vi "Cluster-Find.vi"() -> ()   [LabVIEW 2018]
uses:
  <vilib>/Platform/TimedLoop/XDataNode/timing_clust.ctl
  <vilib>/Platform/TimedLoop/XDataNode/nitl_modes.ctl
  <vilib>/Platform/TimedLoop/XDataNode/wakeup.ctl
  <vilib>/rvi/Emulation/niFpgaSctlEmulationGetInTimedLoop.vi
  <vilib>/rvi/Emulation/niFpgaEmulationReportErrorSimple.vi
  <vilib>/rvi/Emulation/niFpgaGetClockAttributes.vi
  <vilib>/rvi/Emulation/niFpgaCriticalErrorInLSC.vi
  <vilib>/rvi/eio/common/nirviEmuTemplateMethod_errors.vi
  <vilib>/Platform/TimedLoop/XDataNode/XDataNode.xnode
  <vilib>/eio/EIONode/EIONode.xnode
  <vilib>/Platform/TimedLoop/XDataNode/XDNodeRunTimeDep.lvlib
panel:
  out "1":bool[](array[boolean])
  out "2":bool[](array[boolean])
  out "3":bool[](array[boolean])
  out "Nontrivial":i16
  out "4":bool[](array[boolean])
  out "04":i16
  out "03":i16
  out "02":i16
  out "01":i16
  out "clock2":i16
  out "4":i16
  out "3":i16
  out "2":i16
  out "1":i16
  out "Final":bool
  out "2V-ad":bool
  out "2H-ad":bool
  out "1V-ad":bool
  out "1H-ad":bool
  out "SE_Ch4_Rd":bool
  out "SE_Ch3_Rd":bool
  out "SE_Ch2_Rd":bool
  out "SE_Ch1_Rd":bool
  out "clock1":i16
  out "Test":bool
  in  "Probing-Depth":i16
  in  "Stop Button":bool
  in  "2V":i16
  in  "1V":i16
  in  "2H":i16
  in  "1H":i16
  out "Round":u32 format="%^.0e"
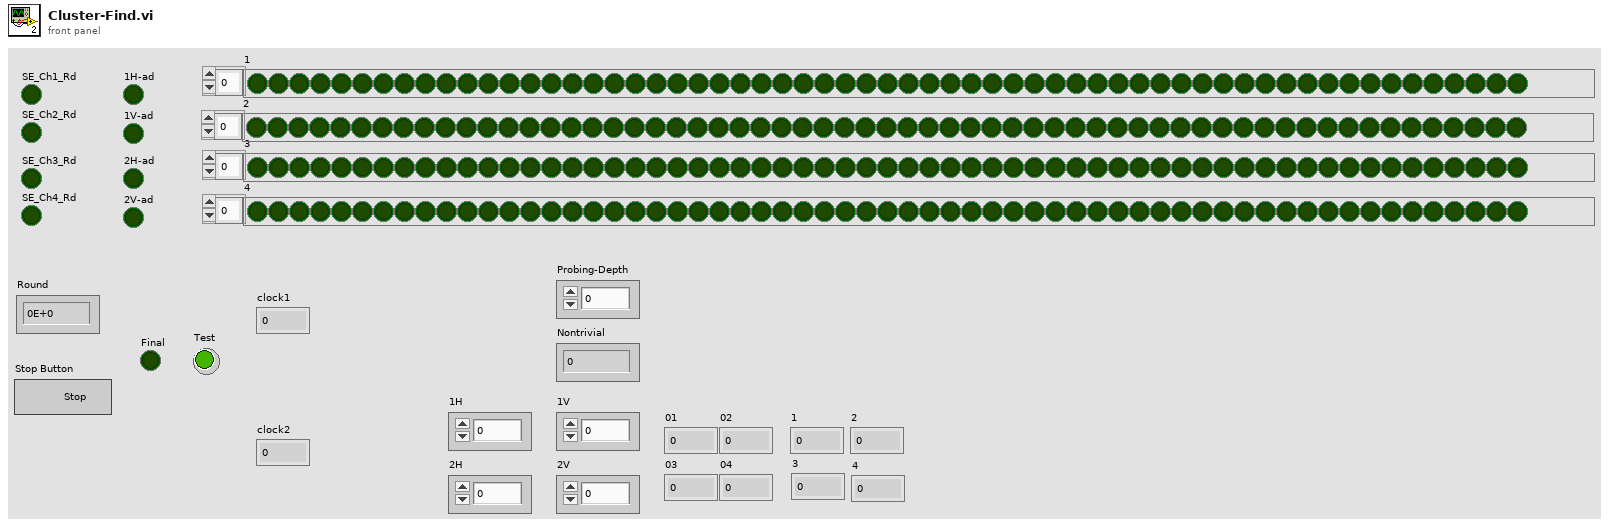
[diagram p1: front panel]
types:
  T1 = typedef "XDNodeRunTimeDep.lvlib/timing_clust.ctl" = cluster{"Expected End [f-1]":u64, "Actual End [f-1]":u64, "Finished Late? [f-1]":bool, "Expected End [i-1]":u64, "Actual End [i-1]":u64, "Finished Late? [i-1]":bool, "Expected Start [i]":u64, "Actual Start [i]":u64, "Expected Start [f]":u64, "Actual Start [f]":u64, "Source Name":string, "Structure Name":string, "Period":i64, "Deadline":i64, "Offset":i64, "Start":i64, "Priority":i32, "Timeout":i32, "Mode":T2, "Wakeup Reason":T3, "Error":errorcluster, "Source Type":string, "Secondary Source Type":string, "Global End Time":u64, "Global Start Time":u64, "Frame Duration":u64, "Iteration Duration":u64, "Assigned CPU":i32, "I/O Scan Engine Mode":u32}
  T2 = typedef "XDNodeRunTimeDep.lvlib/nitl_modes.ctl" = enum32{"No Change", "Process missed periods, maintain original phase", "Discard missed periods, maintain original phase", "Process missed periods, ignore original phase", "Discard missed periods, ignore original phase"}
  T3 = typedef "XDNodeRunTimeDep.lvlib/wakeup.ctl" = enum32{"Normal", "Aborted", "Asynchronous wakeup", "Timing source error", "Timed loop error", "Timeout"}
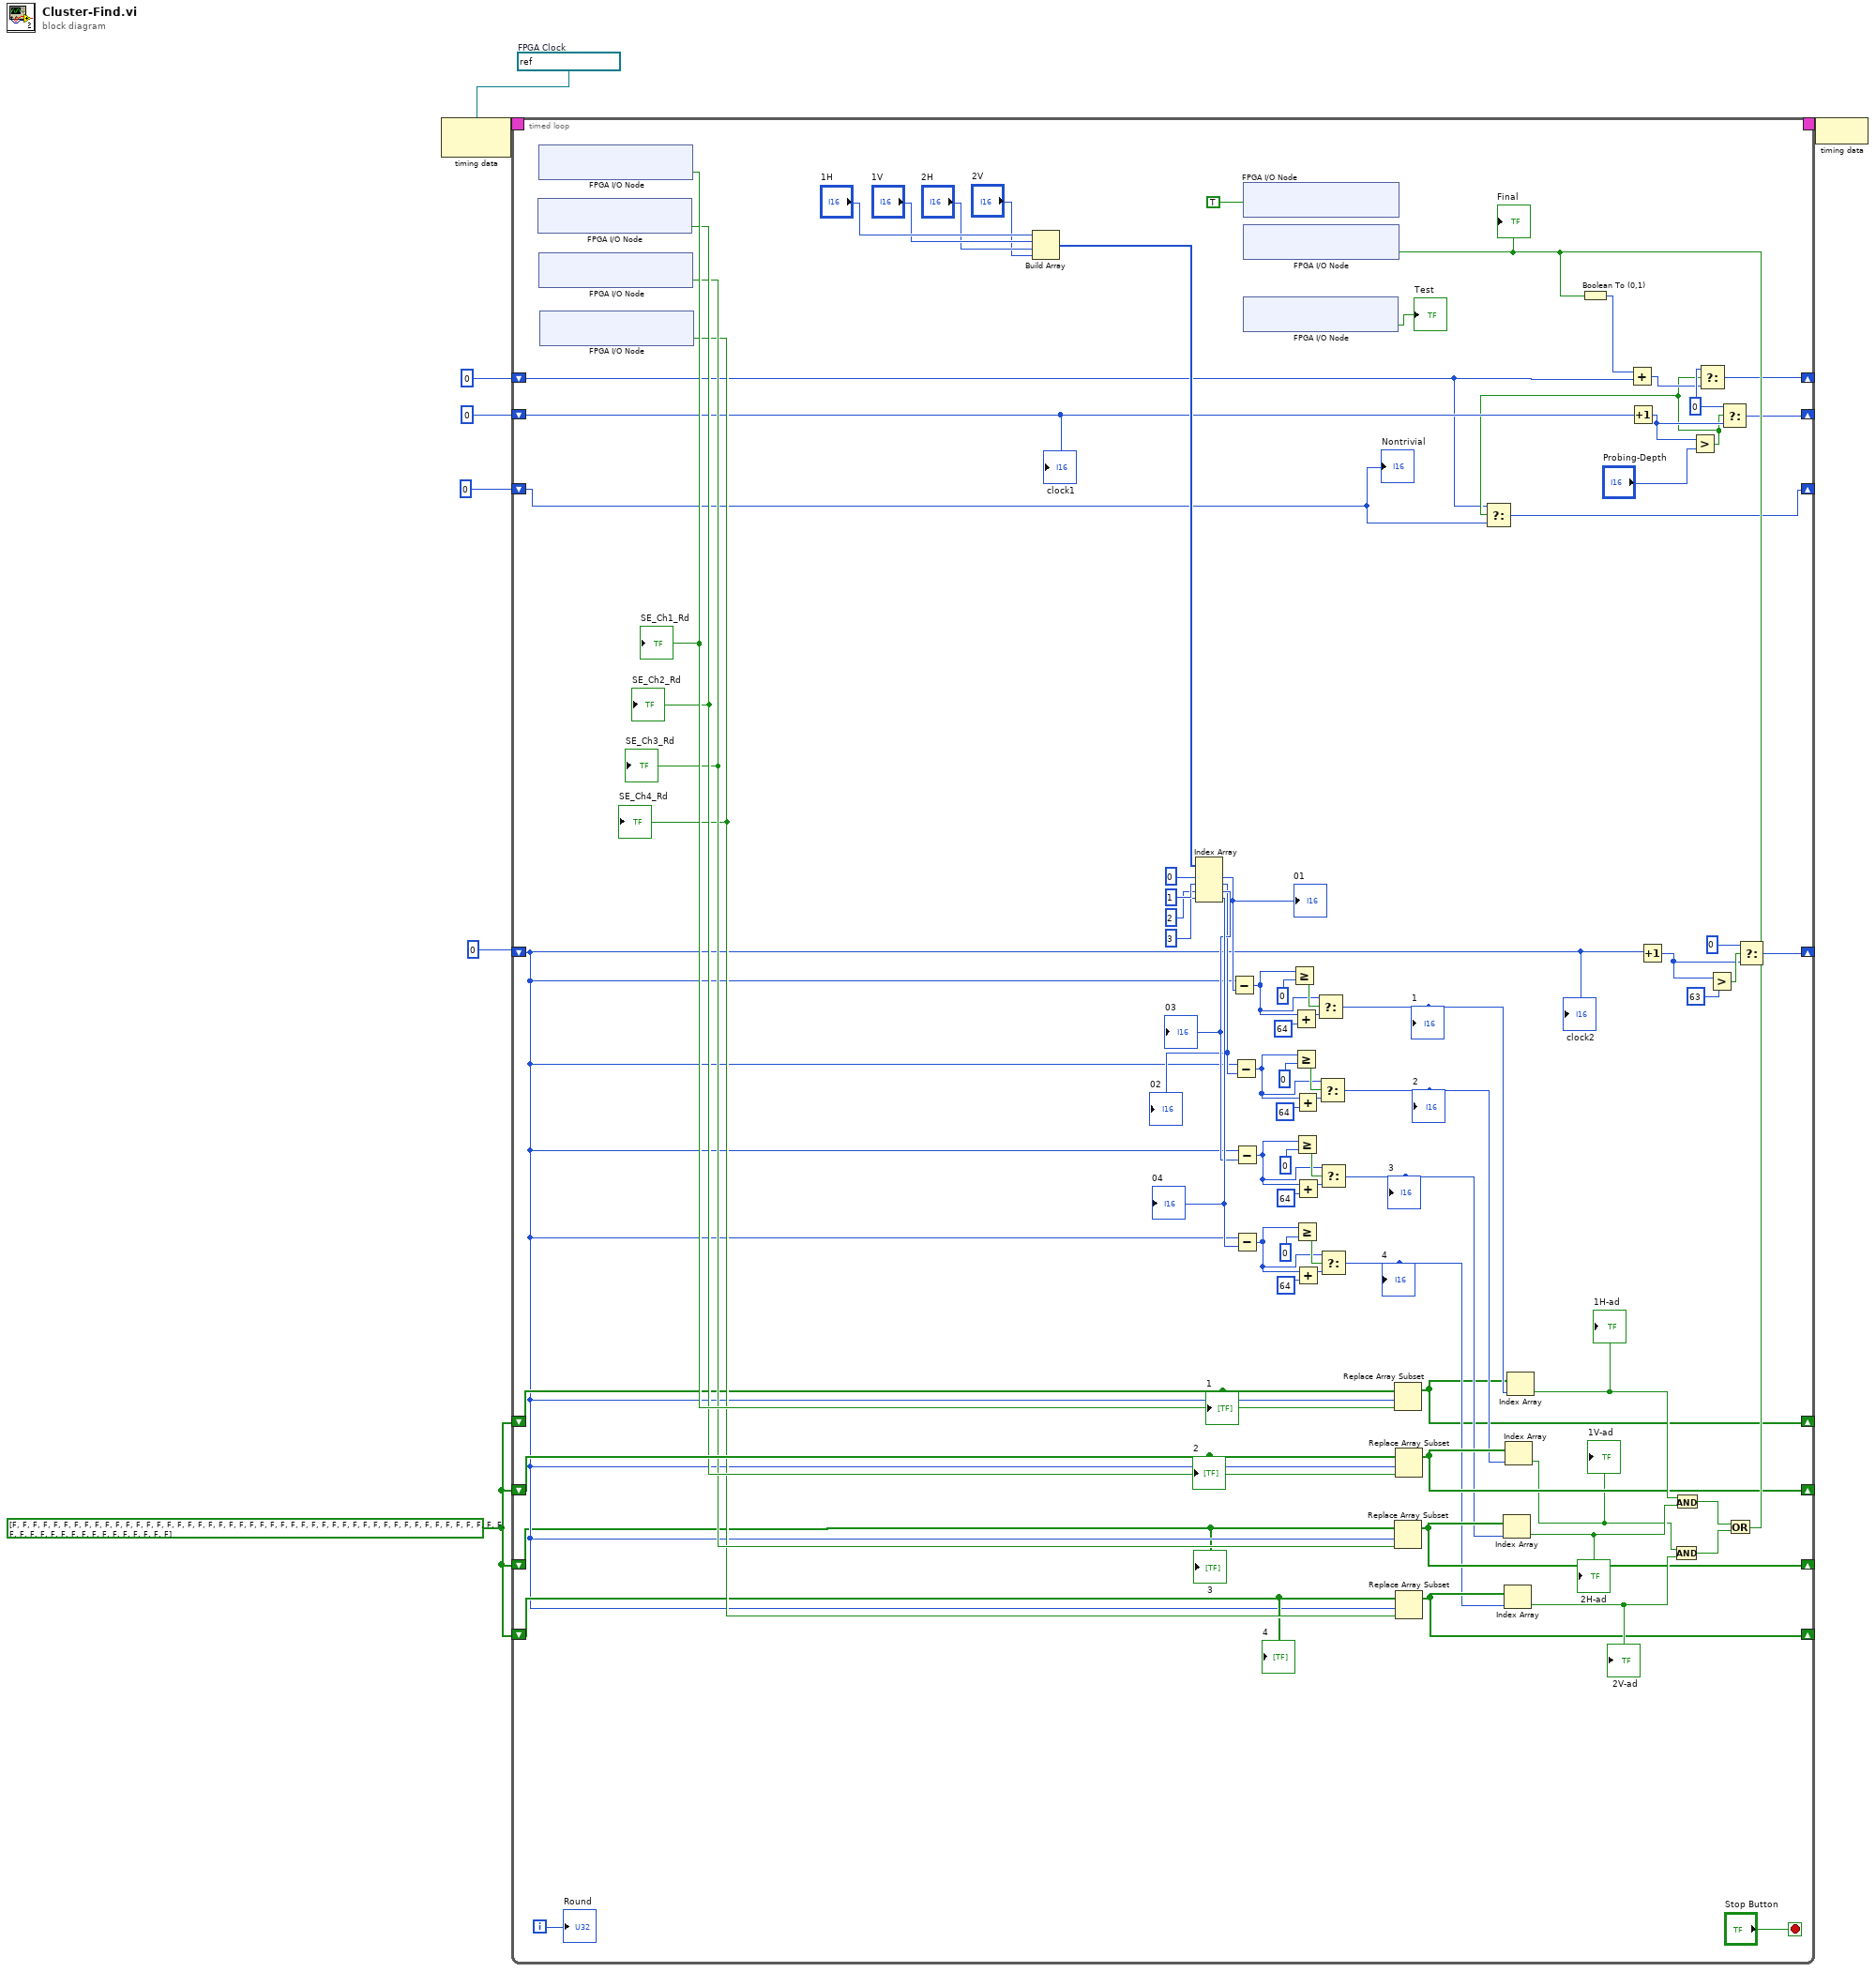
[diagram p0: block diagram]
diagram:
  w5 = bool[] [FALSE, FALSE, FALSE, FALSE, FALSE, FALSE, FALSE, FALSE, FALSE, FALSE, FALSE, FALSE, FALSE, FALSE, FALSE, FALSE, FALSE, FALSE, FALSE, FALSE, FALSE, FALSE, FALSE, FALSE, FALSE, FALSE, FALSE, FALSE, FALSE, FALSE, FALSE, FALSE, FALSE, FALSE, FALSE, FALSE, FALSE, FALSE, FALSE, FALSE, FALSE, FALSE, FALSE, FALSE, FALSE, FALSE, FALSE, FALSE, FALSE, FALSE, FALSE, FALSE, FALSE, FALSE, FALSE, FALSE, FALSE, FALSE, FALSE, FALSE, FALSE, FALSE, FALSE, FALSE]
  w6 = refnum<k21> "200 MHz Clock"  # FPGA Clock
  n1 = node-c288(w6) -> (w8:T1)
  n2 = timed-loop {
    timing: w8 -> [_]
    timing-out: [_] -> w7
    shift-right: [w19] -> _
    shift-left: w5 -> [w15]
    shift-right: [w72] -> _
    shift-left: w5 -> [w73]
    shift-right: [w70] -> _
    shift-left: w5 -> [w13]
    shift-right: [w68] -> _
    shift-left: w5 -> [w16]
    shift-right: [w74] -> _
    shift-left: i16 0 -> [w14]
    shift-right: [w32] -> _
    shift-left: i16 0 -> [w26]
    shift-right: [w27] -> _
    shift-left: i16 0 -> [w10]
    shift-right: [w11] -> _
    shift-left: i16 0 -> [w9]
    i -> [w83]
    stop <- "Stop Button" stop-if-true
    w29 = i16 0
    n3 = xnode "FPGA I/O Node"() -> ("IO Module\\SE_Ch2_Rd"=w71:bool)  [unwired: 1 in, 1 out]
    "SE_Ch2_Rd" <- w71
    n4 = xnode "FPGA I/O Node"() -> ("IO Module\\SE_Ch1_Rd"=w78:bool)  [unwired: 1 in, 1 out]
    "SE_Ch1_Rd" <- w78
    n5 = xnode "FPGA I/O Node"() -> ("IO Module\\SE_Ch3_Rd"=w69:bool)  [unwired: 1 in, 1 out]
    "SE_Ch3_Rd" <- w69
    n6 = xnode "FPGA I/O Node"() -> ("IO Module\\SE_Ch4_Rd"=w67:bool)  [unwired: 1 in, 1 out]
    "SE_Ch4_Rd" <- w67
    n7 = Build Array("1H", "1V", "2H", "2V") -> (w61:i16[])
    n8 = Index Array(array=w61, index #1=i16 0, index #2=i16 1, index #3=i16 2, index #4=i16 3) -> (element #1=w59:i16, element #2=w17:i16, element #3=w18:i16, element #4=w38:i16)
    "01" <- w59
    "02" <- w17
    "03" <- w18
    "04" <- w38
    n9 = Subtract(x=w14, y=w59) -> (x-y=w23:i16)
    n10 = Subtract(x=w14, y=w17) -> (x-y=w22:i16)
    n11 = Subtract(x=w14, y=w18) -> (x-y=w21:i16)
    n12 = Subtract(x=w14, y=w38) -> (x-y=w20:i16)
    n13 = xnode "FPGA I/O Node"("IO Module\\SE_Ch5_Dir"=TRUE) -> ()  [unwired: 1 in, 1 out]
    n14 = xnode "FPGA I/O Node"() -> ("IO Module\\SE_Ch6_Rd"=→"Test":bool)  [unwired: 1 in, 1 out]
    n15 = Greater Or Equal?(x=w23, y=i16 0) -> (x >= y?=w55:bool)
    n16 = Add(x=w23, y=i16 64) -> (x+y=w57:i16)
    n17 = Greater Or Equal?(x=w22, y=i16 0) -> (x >= y?=w48:bool)
    n18 = Greater Or Equal?(x=w21, y=i16 0) -> (x >= y?=w44:bool)
    n19 = Greater Or Equal?(x=w20, y=i16 0) -> (x >= y?=w40:bool)
    n20 = Add(x=w22, y=i16 64) -> (x+y=w50:i16)
    n21 = Add(x=w21, y=i16 64) -> (x+y=w46:i16)
    n22 = Add(x=w20, y=i16 64) -> (x+y=w42:i16)
    n23 = Select(t=w23, s=w55, f=w57) -> (s? t:f=w58:i16)
    "1" <- w58
    n24 = Select(t=w22, s=w48, f=w50) -> (s? t:f=w36:i16)
    "2" <- w36
    n25 = Select(t=w21, s=w44, f=w46) -> (s? t:f=w37:i16)
    "3" <- w37
    n26 = Select(t=w20, s=w40, f=w42) -> (s? t:f=w35:i16)
    "4" <- w35
    n27 = Replace Array Subset(array=w15, new element=w78, index=w14) -> (w19:bool[])
    n28 = Replace Array Subset(array=w13, new element=w69, index=w14) -> (w70:bool[])
    n29 = Replace Array Subset(array=w73, new element=w71, index=w14) -> (w72:bool[])
    n30 = Replace Array Subset(array=w16, new element=w67, index=w14) -> (w68:bool[])
    n31 = Index Array(array=w70, index=w37) -> (element=w80:bool)
    "2H-ad" <- w80
    n32 = Index Array(array=w68, index=w35) -> (element=w81:bool)
    "2V-ad" <- w81
    n33 = Index Array(array=w72, index=w36) -> (element=w24:bool)
    "1V-ad" <- w24
    n34 = Index Array(array=w19, index=w58) -> (element=w82:bool)
    "1H-ad" <- w82
    n35 = Increment(x=w26) -> (x+1=w33:i16)
    n36 = Increment(x=w14) -> (x+1=w66:i16)
    n37 = And(x=w24, y=w81) -> (x .and. y?=w85:bool)
    n38 = And(x=w82, y=w80) -> (x .and. y?=w86:bool)
    n39 = Greater?(x=w33, y="Probing-Depth") -> (0:w12:bool)
    n40 = Select(t=w10, s=w12, f=w9) -> (s? t:f=w11:i16)
    n41 = Greater?(x=w66, y=i16 63) -> (0:w76:bool)
    n42 = Select(t=w29, s=w12, f=w33) -> (s? t:f=w32:i16)
    n43 = Or(x=w86, y=w85) -> (x .or. y?=w79:bool)
    "Final" <- w79
    n44 = xnode "FPGA I/O Node"("IO Module\\SE_Ch5_Wr"=w79) -> ()  [unwired: 1 in, 1 out]
    n45 = Boolean To (0,1)(Boolean=w79) -> (0, 1=w30:i16)
    n46 = Add(x=w30, y=w10) -> (x+y=w28:i16)
    n47 = Select(t=w29, s=w12, f=w28) -> (s? t:f=w27:i16)
    n48 = Select(t=i16 0, s=w76, f=w66) -> (s? t:f=w74:i16)
    "Round" <- w83
    "clock1" <- w26
    "clock2" <- w14
    "4" <- w16
    "Nontrivial" <- w9
    "3" <- w13
    "2" <- w73
    "1" <- w15
  }
  n49 = node-c288(w7) -> ()
